vi "AND16.vi"(2 "B":bool[](array[boolean])=[FALSE, FALSE, FALSE, FALSE, FALSE, FALSE, FALSE, FALSE, FALSE, FALSE, FALSE, FALSE, FALSE, FALSE, FALSE, FALSE], 3 "A":bool[](array[boolean])=[FALSE, FALSE, FALSE, FALSE, FALSE, FALSE, FALSE, FALSE, FALSE, FALSE, FALSE, FALSE, FALSE, FALSE, FALSE, FALSE]) -> (0 "compound":bool, 1 "z":bool[](array[boolean]))   [LabVIEW 2012]
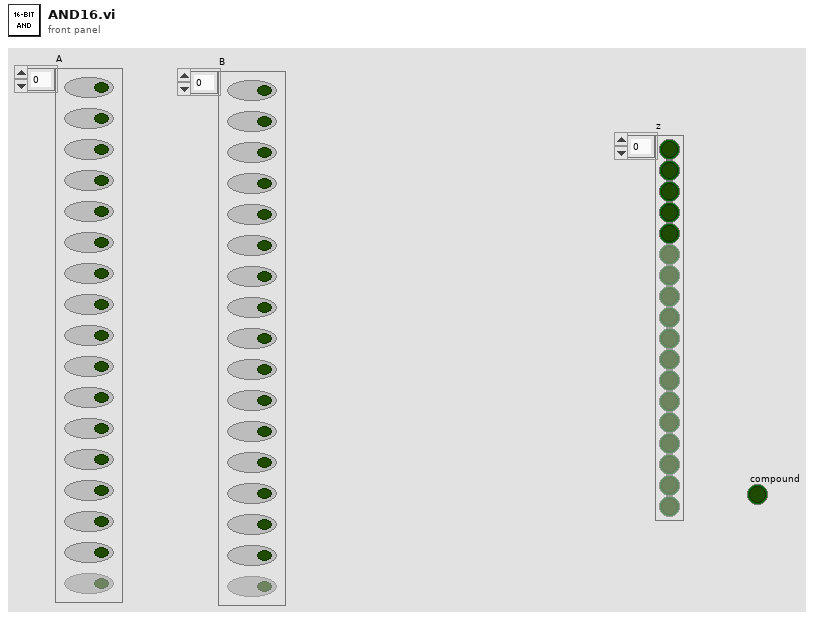
[diagram p1: front panel]
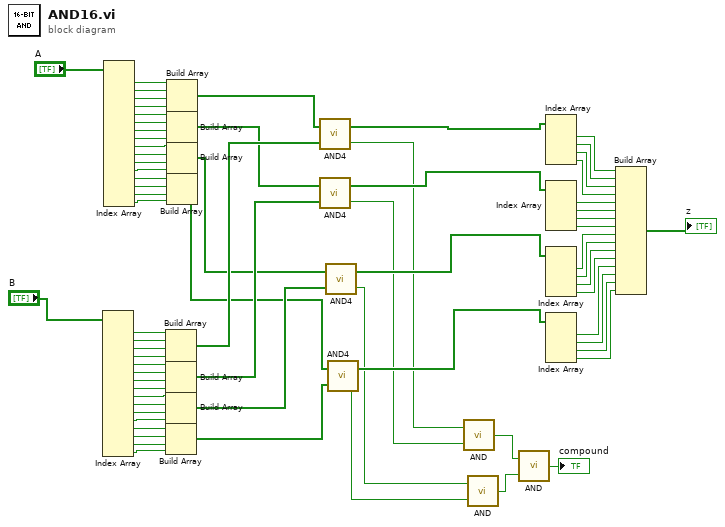
[diagram p0: block diagram]
diagram:
  n1 = Index Array(array="B") -> (element #1=w21:bool, element #2=w22:bool, element #3=w23:bool, element #4=w24:bool, element #5=w25:bool, element #6=w26:bool, element #7=w27:bool, element #8=w28:bool, element #9=w29:bool, element #10=w30:bool, element #11=w31:bool, element #12=w32:bool, element #13=w33:bool, element #14=w34:bool, element #15=w35:bool, element #16=w36:bool)  [unwired: 16 in]
  n2 = Index Array(array="A") -> (element #1=w70:bool, element #2=w69:bool, element #3=w68:bool, element #4=w67:bool, element #5=w66:bool, element #6=w65:bool, element #7=w64:bool, element #8=w63:bool, element #9=w62:bool, element #10=w61:bool, element #11=w60:bool, element #12=w59:bool, element #13=w58:bool, element #14=w57:bool, element #15=w56:bool, element #16=w55:bool)  [unwired: 16 in]
  n3 = Build Array(w21, w22, w23, w24) -> (w18:bool[])
  n4 = Build Array(w25, w26, w27, w28) -> (w16:bool[])
  n5 = Build Array(w29, w30, w31, w32) -> (w14:bool[])
  n6 = Build Array(w33, w34, w35, w36) -> (w12:bool[])
  n7 = Build Array(w70, w69, w68, w67) -> (w19:bool[])
  n8 = Build Array(w66, w65, w64, w63) -> (w17:bool[])
  n9 = Build Array(w62, w61, w60, w59) -> (w15:bool[])
  n10 = Build Array(w58, w57, w56, w55) -> (w13:bool[])
  n11 = call "AND4.vi"("B"=w18, "A"=w19) -> ("compund add"=w7:bool, "z"=w11:bool[])
  n12 = call "AND4.vi"("B"=w16, "A"=w17) -> ("compund add"=w6:bool, "z"=w10:bool[])
  n13 = call "AND4.vi"("B"=w14, "A"=w15) -> ("compund add"=w5:bool, "z"=w9:bool[])
  n14 = call "AND4.vi"("B"=w12, "A"=w13) -> ("compund add"=w4:bool, "z"=w8:bool[])
  n15 = call "AND.vi"("b"=w6, "a"=w7) -> ("x"=w2:bool)
  n16 = call "AND.vi"("b"=w4, "a"=w5) -> ("x"=w3:bool)
  n17 = call "AND.vi"("b"=w3, "a"=w2) -> ("x"=→"compound":bool)
  n18 = Index Array(array=w11) -> (element #1=w54:bool, element #2=w53:bool, element #3=w52:bool, element #4=w51:bool)  [unwired: 4 in]
  n19 = Index Array(array=w10) -> (element #1=w50:bool, element #2=w49:bool, element #3=w48:bool, element #4=w47:bool)  [unwired: 4 in]
  n20 = Index Array(array=w9) -> (element #1=w46:bool, element #2=w45:bool, element #3=w44:bool, element #4=w43:bool)  [unwired: 4 in]
  n21 = Index Array(array=w8) -> (element #1=w42:bool, element #2=w41:bool, element #3=w40:bool, element #4=w39:bool)  [unwired: 4 in]
  n22 = Build Array(w54, w53, w52, w51, w50, w49, w48, w47, w46, w45, w44, w43, w42, w41, w40, w39) -> (→"z":bool[])
